vi "START5ILIKE.vi"() -> ()   [LabVIEW 2024]
uses:
  <vilib>/Utility/file.llb/Read Delimited Spreadsheet (DBL).vi
panel:
  out "Boolean":bool
  in  "Flow Rate Upper Limit":dbl
  in  "Flow Rate Lower Limit":dbl
  in  "stop":bool
  in  "Numeric 2":dbl
  in  "Numeric":dbl
  out "Waveform Chart 3":dbl[](graph)
  out "Waveform Chart 2":dbl[](graph)
  out "Flow Rate":dbl[](graph)
  in  "Color Box":u32(colorbox)
  # "Blood Flow Rate"
  # "LVAD Speed"
  # "Right Heart ?????????"
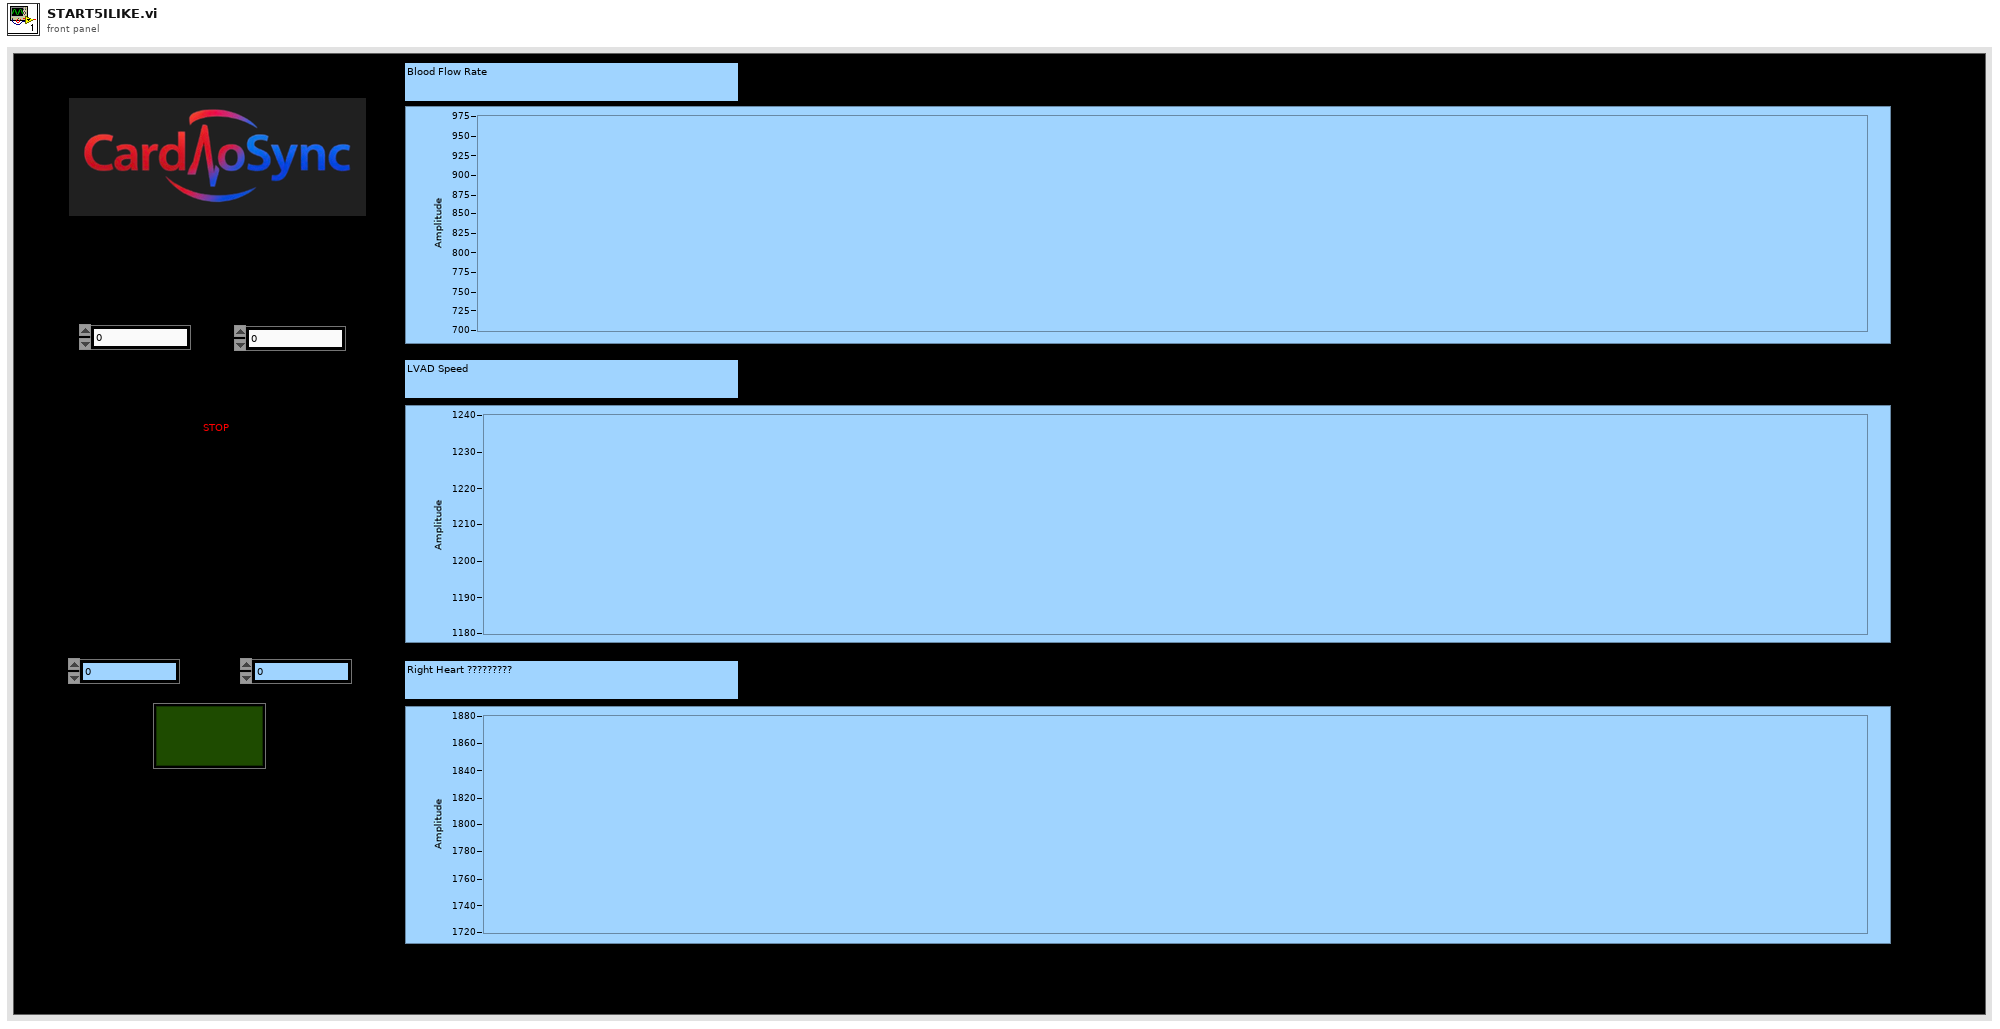
[diagram p1: front panel]
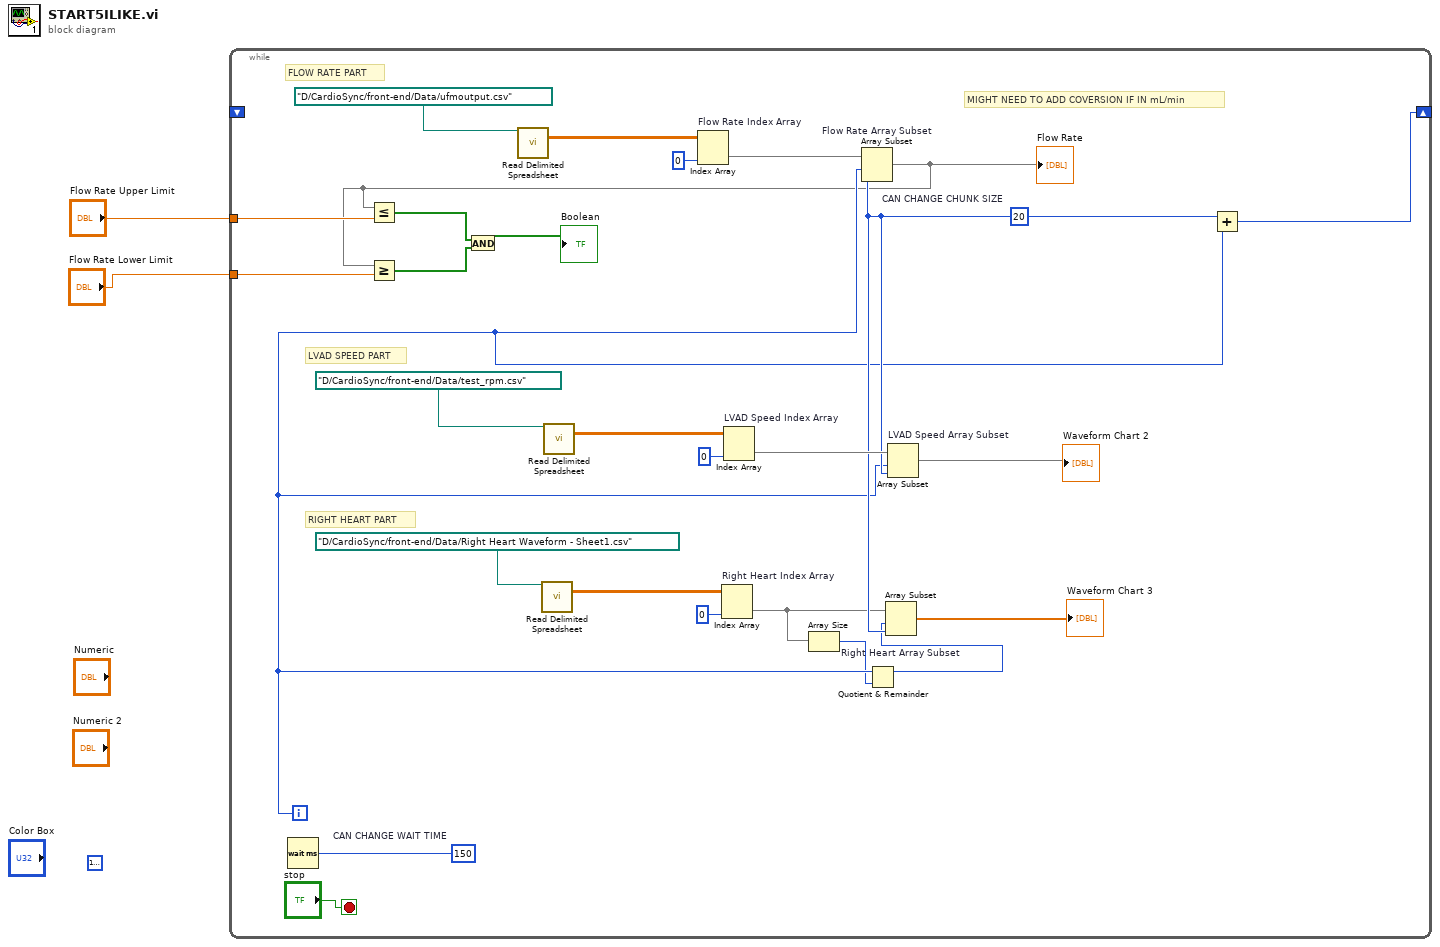
[diagram p0: block diagram]
diagram:
  (unwired) u32 16777228 ("Color Box 2")
  n1 = while {
    shift-right: [w24] -> _
    shift-left: _ -> [_]
    tunnel: "Flow Rate Upper Limit" -> [w8]
    tunnel: "Flow Rate Lower Limit" -> [w7]
    i -> [w11]
    stop <- "stop" stop-if-true
    w25 = u32 150  # CAN CHANGE WAIT TIME
    w17 = 20  # CAN CHANGE CHUNK SIZE
    # "MIGHT NEED TO ADD COVERSION IF IN mL/min"
    # "RIGHT HEART PART"
    # "LVAD SPEED PART"
    # "FLOW RATE PART"
    n2 = Wait (ms)(milliseconds to wait=w25) -> ()  [unwired: 1 out]
    n3 = call-poly <vilib>:"Read Delimited Spreadsheet.vi"("file path (dialog if empty)"=path "D:/CardioSync/front-end/Data/ufmoutput.csv") -> ("all rows"=w27:dbl[][])  [unwired: 9 in, 5 out]
    n4 = call-poly <vilib>:"Read Delimited Spreadsheet.vi"("file path (dialog if empty)"=path "D:/CardioSync/front-end/Data/Right Heart Waveform - Sheet1.csv") -> ("all rows"=w18:dbl[][])  [unwired: 9 in, 5 out]
    n5 = call-poly <vilib>:"Read Delimited Spreadsheet.vi"("file path (dialog if empty)"=path "D:/CardioSync/front-end/Data/test_rpm.csv") -> ("all rows"=w21:dbl[][])  [unwired: 9 in, 5 out]
    n6 = Index Array "Flow Rate Index Array"(array=w27, index (col)=0 ("disabled index (col)")) -> (element=w26:dbl[])  [unwired: 1 in]
    n7 = Index Array "Right Heart Index Array"(array=w18, index (col)=0 ("disabled index (col)")) -> (element=w12:dbl[])  [unwired: 1 in]
    n8 = Index Array "LVAD Speed Index Array"(array=w21, index (col)=0 ("disabled index (col)")) -> (element=w20:dbl[])  [unwired: 1 in]
    n9 = Array Size(array=w12) -> (size(s)=w10:i32)
    n10 = Array Subset "Flow Rate Array Subset"(array=w26, index=w11, length=w17) -> (w5:dbl[])
    "Flow Rate" <- w5
    n11 = Less Or Equal?(x=w5, y=w8) -> (x <= y?=w6:bool[])
    n12 = Greater Or Equal?(x=w5, y=w7) -> (x >= y?=w4:bool[])
    n13 = And(x=w6, y=w4) -> (x .and. y?=→"Boolean":bool[])
    n14 = Quotient & Remainder(x=w11, y=w10) -> (x-y*floor(x/y)=w9:i32)  [unwired: 1 out]
    n15 = Array Subset "Right Heart Array Subset"(array=w12, index=w9, length=w17) -> (→"Waveform Chart 3":dbl[])
    n16 = Array Subset "LVAD Speed Array Subset"(array=w20, index=w11, length=w17) -> (→"Waveform Chart 2":dbl[])
    n17 = Add(x=w17, y=w11) -> (x+y=w24:i32)
  }
